vi "Look in Map.vi"(8 "error in":errorcluster, 10 "Key":string, 11 "Map":map{string, i32}(c390)) -> (0 "error out":errorcluster, 3 "Value":i32)   [LabVIEW 2023]
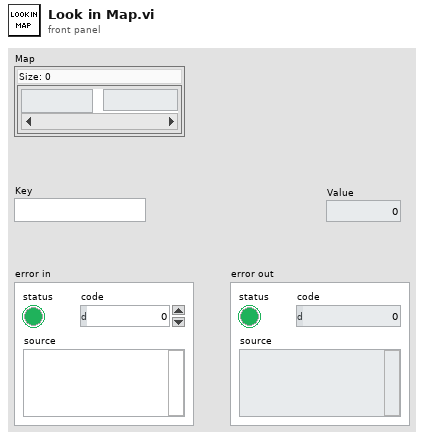
[diagram p1: front panel]
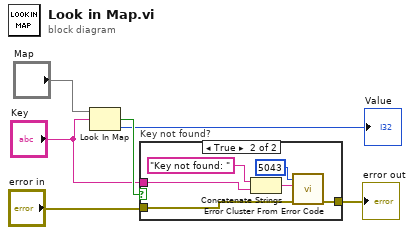
[diagram p0: block diagram]
diagram:
  n1 = Look In Map(map="Map", key="Key") -> (key not found?=w4:bool, value=→"Value":i32)  [unwired: 1 in]
  n2 = case "Key not found?" shown="True" w4 {
    tunnel: "error in" -> [w7 w8]
    tunnel: [w7 w13] -> w3
    tunnel: "Key" -> [_ w9]
    frame False {
    }
    frame True {
      n3 = Concatenate Strings("Key not found: " ("string"), w9) -> (w11:string)
      n4 = call <vilib>:"Error Cluster From Error Code.vi"("error in (no error)"=w8, "error message (\"\")"=w11, "error code (0)"=5043) -> ("error out"=w13:errorcluster)  [unwired: 6 in]
    }
  }
  "error out" <- w3
